vi "Read transaction.vi"(8 "error in (no error)":errorcluster, 11 "DbConnection in":refnum<class "ORM_DBC_dotNet.lvclass">) -> (0 "error out":errorcluster, 2 "BeginTransaction":refnum<k24>, 3 "DbConnection out":refnum<class "ORM_DBC_dotNet.lvclass">)   [LabVIEW 2020, in "ORM_DBC_dotNet.lvlib" / "ORM_DBC_dotNet.lvclass"]
uses:
  ORM_DBC_dotNet.lvclass
  System.Data
  ORM_DBC_dotNet.lvclass/ORM_DBC_dotNet.ctl
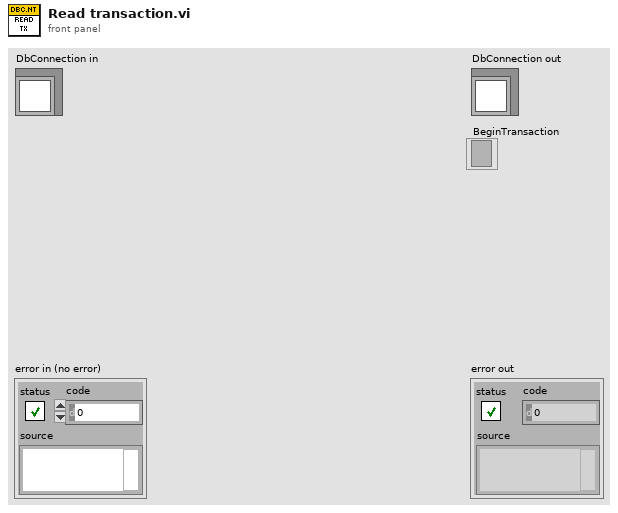
[diagram p1: front panel]
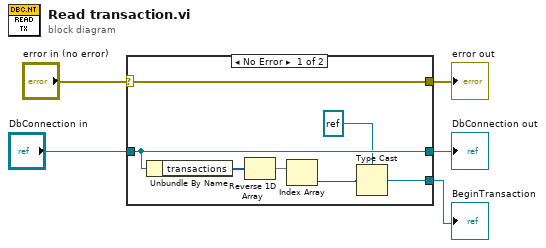
[diagram p0: block diagram]
diagram:
  n1 = case shown="No Error" "error in (no error)" {
    selector: "error in (no error)" -> [w12 w13]
    tunnel: [w12 w13] -> w4
    tunnel: [w11 w14] -> w2
    tunnel: "DbConnection in" -> [w11 w14]
    tunnel: [w6 _] -> w1
    frame No Error {
      n2 = Unbundle By Name(w11) -> ("transactions"=w10:u64[])
      n3 = Reverse 1D Array(array=w10) -> (reversed array=w9:u64[])
      n4 = Index Array(array=w9) -> (element=w8:u64)  [unwired: 1 in]
      n5 = Type Cast(type=refnum<k24> refnum ("BeginTransaction"), x=w8) -> (*(type *) &x=w6:refnum<k24>)
    }
    frame Error {
    }
  }
  "error out" <- w4
  "DbConnection out" <- w2
  "BeginTransaction" <- w1
